vi "_UpdateDisplay.vi"(9 "Action in":T4 caption="Action", 10 "Display State In in":T1 caption="State", 11 "Data In in":T5) -> (1 "Action out":T4 caption="Action", 2 "Display State In out":T1 caption="State", 3 "Data In out":T5)   [LabVIEW 2013, in "UI_TimeSelector.xctl"]
uses:
  UI_TimeSelector.xctl
  Data.ctl
  <vilib>/_xctls/Action.ctl
  State.ctl
  Typedefs/INTERNAL-DATA.ctl
  Interface/DEF-Mode.ctl
  <vilib>/_xctls/XControlSupport.lvlib
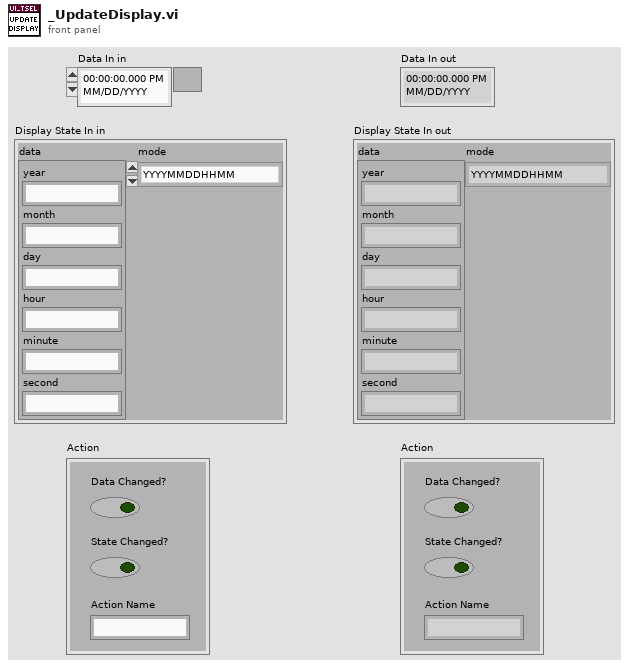
[diagram p1: front panel]
types:
  T1 = typedef "UI_TimeSelector.xctl/State.ctl" = cluster{"data":T2, "mode":T3}
  T2 = typedef "UI_TimeSelector.xctl/INTERNAL-DATA.ctl" = cluster{"year":string, "month":string, "day":string, "hour":string, "minute":string, "second":string}
  T3 = typedef "UI_TimeSelector.xctl/DEF-Mode.ctl" = enum16{"YYYYMMDDHHMM", "YYYYMMDDHHMMSS", "YYYY", "YYYYMM", "YYYYMMDD", "HHMM", "HHMMSS"}
  T4 = typedef "XControlSupport.lvlib/Action.ctl" = cluster{"Data Changed?":bool, "State Changed?":bool, "Action Name":string}
  T5 = typedef "UI_TimeSelector.xctl/Data.ctl" = timestamp
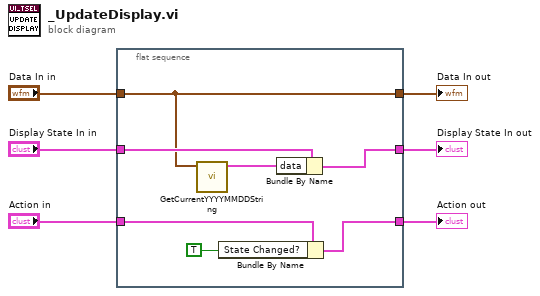
[diagram p0: block diagram]
diagram:
  n1 = flat-sequence {
    tunnel: "Display State In in" -> [w13]
    tunnel: [w12] -> w2
    tunnel: [w11] -> w3
    tunnel: "Action in" -> [w10]
    tunnel: "Data In in" -> [w7]
    tunnel: [w7] -> w6
    frame #0 {
      n2 = call "GetCurrentYYYYMMDDString.vi"("displayTime"=w7) -> ("data"=w8:T2)  [unwired: 10 in]
      n3 = Bundle By Name(cluster=w10, "State Changed?"=TRUE) -> (w11:T4)
      n4 = Bundle By Name(cluster=w13, "data"=w8) -> (w12:T1)
    }
  }
  "Data In out" <- w6
  "Action out" <- w3
  "Display State In out" <- w2
